vi "SQL_SelectArray.vi"(9 "SQL query":string, 11 "ConnectionDSN":string) -> (1 "data":string[](array[string]))   [LabVIEW 2017]
uses:
  <vilib>/addons/database/Connection.llb/DB Tools Open Connec (String).vi
  <vilib>/addons/database/Connection.llb/Conn Execute.vi
  <vilib>/addons/database/Recordset.llb/Rec Fetch Recordset Data (R).vi
  <vilib>/addons/database/_DB Variant To Data/Database Variant To Data.xnode
  <vilib>/addons/database/NI_Database_API.lvlib
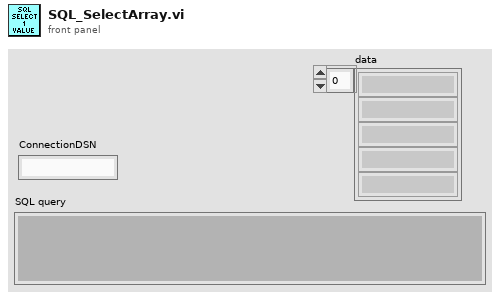
[diagram p1: front panel]
types:
  T1 = typedef "NI_Database_API.lvlib/Conn ObjectReference.ctl" = refnum<k1>
  T2 = typedef "NI_Database_API.lvlib/Rec ObjectReference.ctl" = refnum<k1>
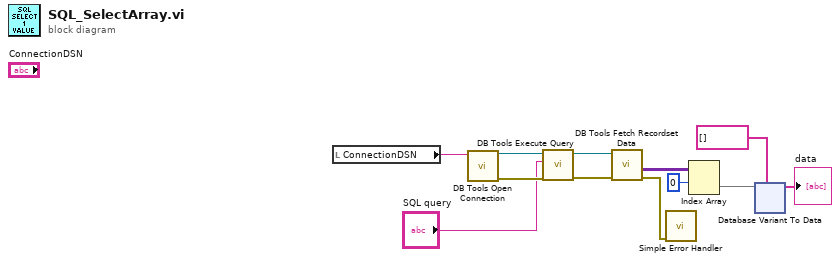
[diagram p0: block diagram]
diagram:
  n1 = local read "ConnectionDSN"() -> (w12:string)
  n2 = call-poly <vilib>:"DB Tools Open Connection.vi"("connection information"=w12) -> ("error out"=w9:errorcluster, "connection reference"=w11:T1)  [unwired: 7 in]
  n3 = call-poly <vilib>:"DB Tools Execute Query.vi"("error in (no error)"=w9, "SQL query"="SQL query", "connection reference"=w11) -> ("error out"=w8:errorcluster, "recordset reference"=w10:T2)  [unwired: 5 in]
  n4 = call-poly <vilib>:"DB Tools Fetch Recordset Data.vi"("error in (no error)"=w8, "recordset reference"=w10) -> ("error out"=w4:errorcluster, "recordset data"=w6:variant[][])  [unwired: 3 in, 1 out]
  n5 = call <vilib>:"Simple Error Handler.vi"("error in (no error)"=w4) -> ()  [unwired: 4 in, 5 out]
  n6 = Index Array(array=w6, index (row)=0) -> (element=w3:variant[])  [unwired: 1 in]
  n7 = xnode "Database Variant To Data"("database variant"=w3, "type"=string[] []) -> ("data"=→"data":string[])  [unwired: 1 in, 1 out]
